vi "Set HLAfloat64BE.vi"(11 "eu data in":dbl[](array[numeric])) -> (1 "valid":bool=TRUE, 3 "raw data out":u8[](array[numeric]))   [LabVIEW 2019, in "HLA Data Conversion.lvlib"]
uses:
  HLA Data Conversion.lvlib
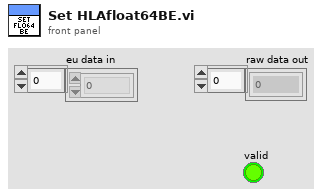
[diagram p1: front panel]
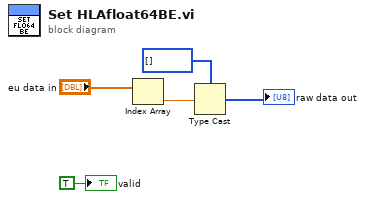
[diagram p0: block diagram]
diagram:
  n1 = Index Array(array="eu data in") -> (element=w3:dbl)  [unwired: 1 in]
  n2 = Type Cast(type=u8[] [] ("raw data out"), x=w3) -> (*(type *) &x=→"raw data out":u8[])
  "valid" <- TRUE
